vi "Find Mouse Down Option.vi"(8 "error in":errorcluster, 10 "Menu Position":T2, 11 "Mouse DownCoords":T1) -> (0 "error out":errorcluster, 3 "Button Index":u32)   [LabVIEW 2019]
doc: "All Rights Reserved © 2017 SyncSols"
uses:
  <vilib>/Utility/miscctls.llb/LVPositionTypeDef.ctl
  <vilib>/Utility/miscctls.llb/LVPoint32TypeDef.ctl
  <vilib>/Utility/miscctls.llb/LVBoundsTypeDef.ctl
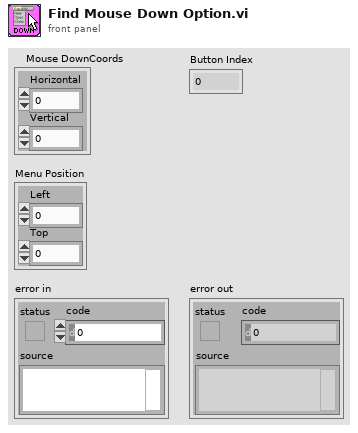
[diagram p1: front panel]
types:
  T1 = typedef "LVPoint32TypeDef.ctl" = cluster{"Horizontal":i32, "Vertical":i32}
  T2 = typedef "LVPositionTypeDef.ctl" = cluster{"Left":i32, "Top":i32}
  T3 = typedef "LVBoundsTypeDef.ctl" = cluster{"Width":u32, "Height":u32}
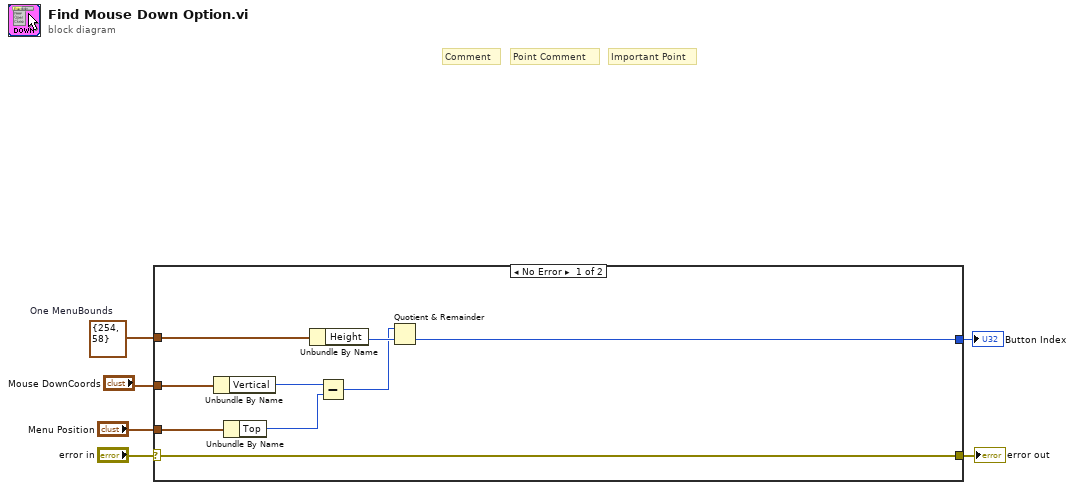
[diagram p0: block diagram]
diagram:
  w2 = T3 {"Width"=254, "Height"=58}  # One MenuBounds
  # "Important Point"
  # "Point Comment"
  # "Comment"
  n1 = case shown="No Error" "error in" {
    selector: "error in" -> [w15 w16]
    tunnel: [w15 w16] -> w6
    tunnel: "Menu Position" -> [w14 _]
    tunnel: "Mouse DownCoords" -> [w13 _]
    tunnel: [w8 _] -> w1
    tunnel: w2 -> [w7 _]
    frame No Error {
      n2 = Unbundle By Name(w13) -> ("Vertical"=w12:i32)
      n3 = Unbundle By Name(w14) -> ("Top"=w11:i32)
      n4 = Unbundle By Name(w7) -> ("Height"=w10:u32)
      n5 = Subtract(x=w12, y=w11) -> (x-y=w9:i32)
      n6 = Quotient & Remainder(x=w9, y=w10) -> (floor(x/y)=w8:u32)  [unwired: 1 out]
    }
    frame Error {
    }
  }
  "error out" <- w6
  "Button Index" <- w1
